vi "OAT Estimate Max Order.vi"(5 "reset? (True)":bool=TRUE, 10 "speed profile in":T1 {"speed [RPM]" format="%.2f"; "time [s]" format="%.2f"}, 11 "scaled signal [EU] in":waveform(dbl)) -> (0 "max possible order":dbl format="%.2f", 1 "max suggested order":dbl format="%.2f", 2 "speed profile out":T1 {"speed [RPM]" format="%.2f"; "time [s]" format="%.2f"}, 3 "scaled signal [EU] out":waveform(dbl))   [LabVIEW 2017, in "SoundVib_Resampling.lvlib"]
uses:
  <vilib>/addons/Sound and Vibration/Order Analysis/Resample Order Tracking/SoundVib_Resampling.lvlib
  <vilib>/addons/Sound and Vibration/Order Analysis/Tach Process/SubVIs/speed profile.ctl
  <vilib>/Waveform/WDTOps.llb/WDT Waveform Duration DBL.vi
  <vilib>/addons/Sound and Vibration/Order Analysis/Tach Process/SoundVib_TachProcess.lvlib
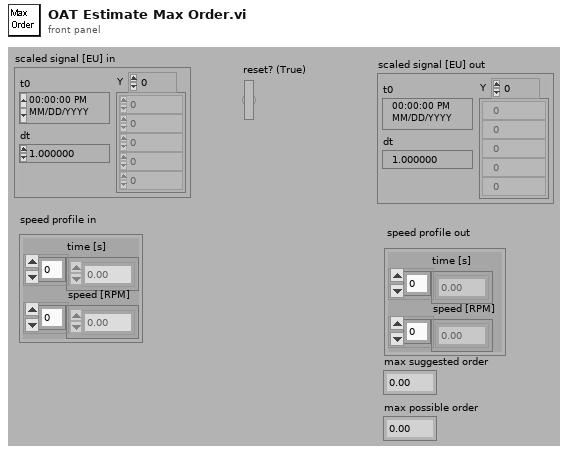
[diagram p1: front panel]
types:
  T1 = typedef "SoundVib_TachProcess.lvlib/speed profile.ctl" = cluster{"time [s]":dbl[], "speed [RPM]":dbl[]}
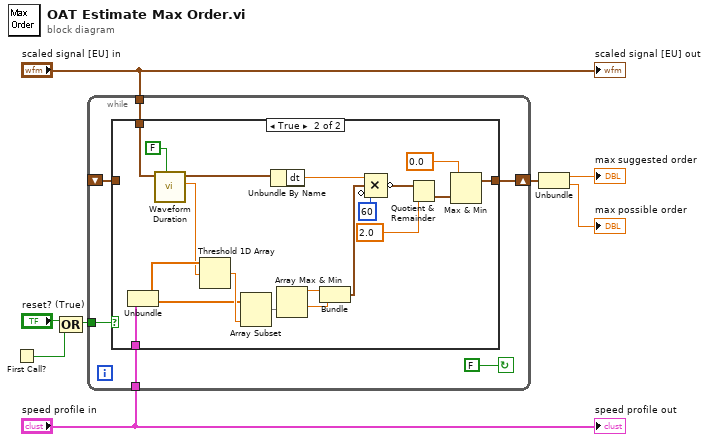
[diagram p0: block diagram]
diagram:
  n1 = First Call?() -> (First Call?: T/F=w3:bool)
  n2 = Compound Arithmetic op=OR("reset? (True)", w3) -> (w2:bool)
  n3 = while {
    tunnel: "scaled signal [EU] in" -> [w14]
    tunnel: "speed profile in" -> [w13]
    tunnel: w2 -> [w11]
    shift-right: [w10] -> w1
    shift-left: _ -> [w9]
    stop <- FALSE continue-if-true
    n4 = case shown="True" w11 {
      tunnel: w14 -> [_ w22]
      tunnel: w13 -> [_ w28]
      tunnel: [w15 w24] -> w10
      tunnel: w9 -> [w15 _]
      frame False {
      }
      frame True {
        n5 = Unbundle(w28) -> ("time [s]"=w20:dbl[], "speed [RPM]"=w17:dbl[])
        n6 = call-poly <vilib>:"Waveform Duration.vi"("open interval? (T)"=FALSE, "waveform in"=w22) -> ("duration"=w19:dbl, "waveform out"=w23:waveform(dbl))  [unwired: 7 in, 1 out]
        n7 = Threshold 1D Array(2:w19, 3:w20) -> (0:w18:dbl)  [unwired: 1 in]
        n8 = Array Subset(array=w17, length=w18) -> (w16:dbl[])  [unwired: 1 in]
        n9 = Unbundle By Name(w23) -> ("dt"=w29:dbl)
        n10 = Array Max & Min(array=w16) -> (max value=w27:dbl, min value=w26:dbl)  [unwired: 2 out]
        n11 = Bundle(w27, w26) -> (w25:cluster{dbl, dbl})  [unwired: 1 in]
        n12 = Compound Arithmetic op=MULTIPLY(w29, w25, invert 60) -> (invert w31:cluster{dbl, dbl})
        n13 = Quotient & Remainder(x=w31, y=2.0) -> (floor(x/y)=w33:cluster{dbl, dbl})  [unwired: 1 out]
        n14 = Max & Min(x=0.0, y=w33) -> (max(x,y)=w24:cluster{dbl, dbl})  [unwired: 1 out]
      }
    }
  }
  n15 = Unbundle(w1) -> (→"max suggested order":dbl, →"max possible order":dbl)
  "scaled signal [EU] out" <- "scaled signal [EU] in"
  "speed profile out" <- "speed profile in"
